vi "createCommand.vi"(8 "error in (no error)":errorcluster, 10 "commandValue":T1=enum."disable", 11 "CommandFactory in":refnum<class "CommandFactory.lvclass">) -> (0 "error out":errorcluster, 2 "command":refnum<class "Command.lvclass">, 3 "CommandFactory out":refnum<class "CommandFactory.lvclass">)   [LabVIEW 2016, in "CommandFactory.lvclass"]
uses:
  CommandFactory.lvclass
  Commands/Disable/disable.lvclass
  Commands/Enable/enable.lvclass
  Commands/Exit/exit.lvclass
  Commands/GoToStandby/standby.lvclass
  Commands/OnInterrupt/OnInterrupt.lvclass
  Commands/Start/start.lvclass
  Commands/OnIncomingMessagingError/OnIncomingMessagingError.lvclass
  Commands/OnHeartbeat/OnHeartbeat.lvclass
  Commands/CaptureSpectImage/captureSpectImage.lvclass
  home/harini/tcs/ts_sedspectrometer/CommandThisComponent/CommandThisComponent.lvclass
  home/harini/tcs/ts_sedspectrometer/ComponentTemplateCore/ComponentModel/ComponentModel/Command/Command.lvclass
  CommandThisComponent/CommandThisComponent.lvclass
  ComponentTemplateCore/ComponentModel/ComponentModel/Command/Command.lvclass
  Typedefs/CommandValue.ctl
  Typedefs/SEDSpectrometerTypedefs.lvlib
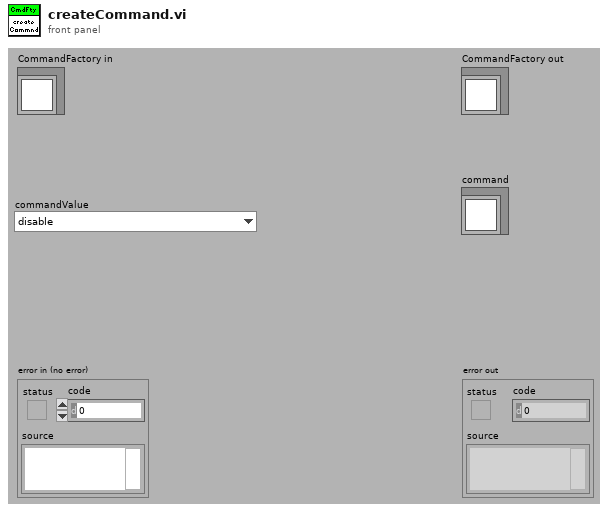
[diagram p1: front panel]
types:
  T1 = typedef "SEDSpectrometerTypedefs.lvlib/CommandValue.ctl" = enum16{"clearError", "disable", "enable", "exit", "GoToStandby", "OnHeartbeat", "OnIncomingMessagingError", "OnInterrupt", "start", "captureSpectImage", "setSpectTempSetpoint", "stopImageCapture"}
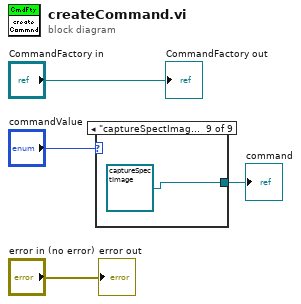
[diagram p0: block diagram]
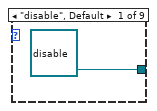
[diagram p2: hidden frame]
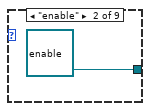
[diagram p3: hidden frame]
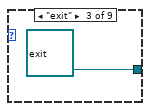
[diagram p4: hidden frame]
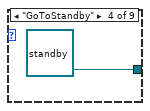
[diagram p5: hidden frame]
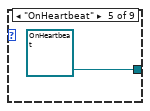
[diagram p6: hidden frame]
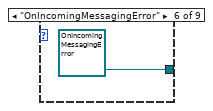
[diagram p7: hidden frame]
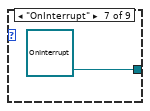
[diagram p8: hidden frame]
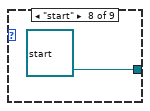
[diagram p9: hidden frame]
diagram:
  n1 = case shown="\"captureSpectImage\"" "commandValue" {
    tunnel: [refnum<class "disable.lvclass"> refnum ("Commands.lvlib:Disable.lvclass") refnum<class "enable.lvclass"> refnum ("Commands.lvlib:Enable.lvclass") refnum<class "exit.lvclass"> refnum ("Commands.lvlib:Exit.lvclass") refnum<class "standby.lvclass"> refnum ("Commands.lvlib:GoToStandby.lvclass") refnum<class "OnHeartbeat.lvclass"> refnum ("Commands.lvlib:OnHeartbeat.lvclass") refnum<class "OnIncomingMessagingError.lvclass"> refnum ("Commands.lvlib:OnIncomingMessagingError.lvclass") refnum<class "OnInterrupt.lvclass"> refnum ("Commands.lvlib:OnInterrupt.lvclass") refnum<class "start.lvclass"> refnum ("Commands.lvlib:Start.lvclass") refnum<class "captureSpectImage.lvclass"> refnum ("Commands.lvlib:CaptureSpectImage.lvclass")] -> w1
    frame "disable", Default {
    }
    frame "enable" {
    }
    frame "exit" {
    }
    frame "GoToStandby" {
    }
    frame "OnHeartbeat" {
    }
    frame "OnIncomingMessagingError" {
    }
    frame "OnInterrupt" {
    }
    frame "start" {
    }
    frame "captureSpectImage" {
    }
  }
  "command" <- w1
  "error out" <- "error in (no error)"
  "CommandFactory out" <- "CommandFactory in"
